vi "Get IConfiguration.vi"(8 "error in":errorcluster, 11 "IHas Configuration in":refnum<class "IHas Configuration.lvclass">) -> (0 "error out":errorcluster, 2 "IConfiguration":refnum<class "IConfiguration.lvclass">, 3 "IHas Configuration out":refnum<class "IHas Configuration.lvclass">)   [LabVIEW 2024, in "IHas Configuration.lvclass"]
uses:
  IHas Configuration.lvclass
  IConfiguration/IConfiguration.lvclass
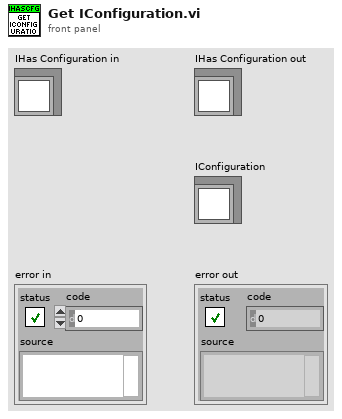
[diagram p1: front panel]
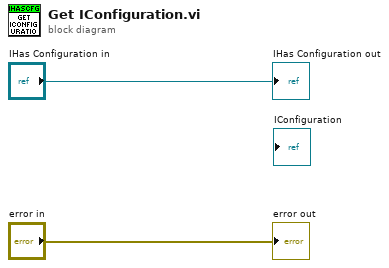
[diagram p0: block diagram]
diagram:
  "error out" <- "error in"
  "IHas Configuration out" <- "IHas Configuration in"
